vi "hysteresis_fxp_16_5.vi"(8 "N_hyst":u8=3, 11 "uk_in":fxp<+/-,16,5>) -> (3 "Hinv(uk)":fxp<+/-,32,10>)   [LabVIEW 2017]
uses:
  <vilib>/Platform/TimedLoop/XDataNode/timing_clust.ctl
  <vilib>/Platform/TimedLoop/XDataNode/nitl_modes.ctl
  <vilib>/Platform/TimedLoop/XDataNode/wakeup.ctl
  <vilib>/rvi/Emulation/niFpgaSctlEmulationGetInTimedLoop.vi
  <vilib>/rvi/Emulation/niFpgaEmulationReportErrorSimple.vi
  <vilib>/rvi/Emulation/niFpgaGetClockAttributes.vi
  <vilib>/rvi/Emulation/niFpgaCriticalErrorInLSC.vi
  <vilib>/rvi/Memory/Memory_Emulation/nirvimemoryFastEmulation.vi
  <vilib>/rvi/Memory/Memory_Emulation/nirvimemoryEmulation.vi
  <vilib>/rvi/Emulation/niFpgaEmulationIsFPGAContextNoSignature.vi
  <vilib>/rvi/DataTransferAndStorage/Container/Common/niFpgaContainerGetUniqueNameForEmu.vi
  <vilib>/rvi/Emulation/niFpgaProcessEmulError.vi
  <vilib>/rvi/errors/nirviReportUnexpectedCaseInternalError (U32).vi
  <vilib>/Platform/TimedLoop/XDataNode/XDataNode.xnode
  <vilib>/rvi/DataTransferAndStorage/Container/XNode/niFpgaContainer.xnode
  <vilib>/rvi/FXPMathLib/FxpSub/XNode/nifxpmath_Sub.xnode
  <vilib>/rvi/FXPMathLib/FxpAdd/XNode/nifxpmath_Add.xnode
  <vilib>/Platform/TimedLoop/XDataNode/XDNodeRunTimeDep.lvlib
  <vilib>/rvi/FXPMathLib/sim/FxpSim.dll
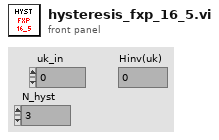
[diagram p1: front panel]
types:
  T1 = typedef "XDNodeRunTimeDep.lvlib/timing_clust.ctl" = cluster{"Expected End [f-1]":u64, "Actual End [f-1]":u64, "Finished Late? [f-1]":bool, "Expected End [i-1]":u64, "Actual End [i-1]":u64, "Finished Late? [i-1]":bool, "Expected Start [i]":u64, "Actual Start [i]":u64, "Expected Start [f]":u64, "Actual Start [f]":u64, "Source Name":string, "Structure Name":string, "Period":i64, "Deadline":i64, "Offset":i64, "Start":i64, "Priority":i32, "Timeout":i32, "Mode":T2, "Wakeup Reason":T3, "Error":errorcluster, "Source Type":string, "Secondary Source Type":string, "Global End Time":u64, "Global Start Time":u64, "Frame Duration":u64, "Iteration Duration":u64, "Assigned CPU":i32, "I/O Scan Engine Mode":u32}
  T2 = typedef "XDNodeRunTimeDep.lvlib/nitl_modes.ctl" = enum32{"No Change", "Process missed periods, maintain original phase", "Discard missed periods, maintain original phase", "Process missed periods, ignore original phase", "Discard missed periods, ignore original phase"}
  T3 = typedef "XDNodeRunTimeDep.lvlib/wakeup.ctl" = enum32{"Normal", "Aborted", "Asynchronous wakeup", "Timing source error", "Timed loop error", "Timeout"}
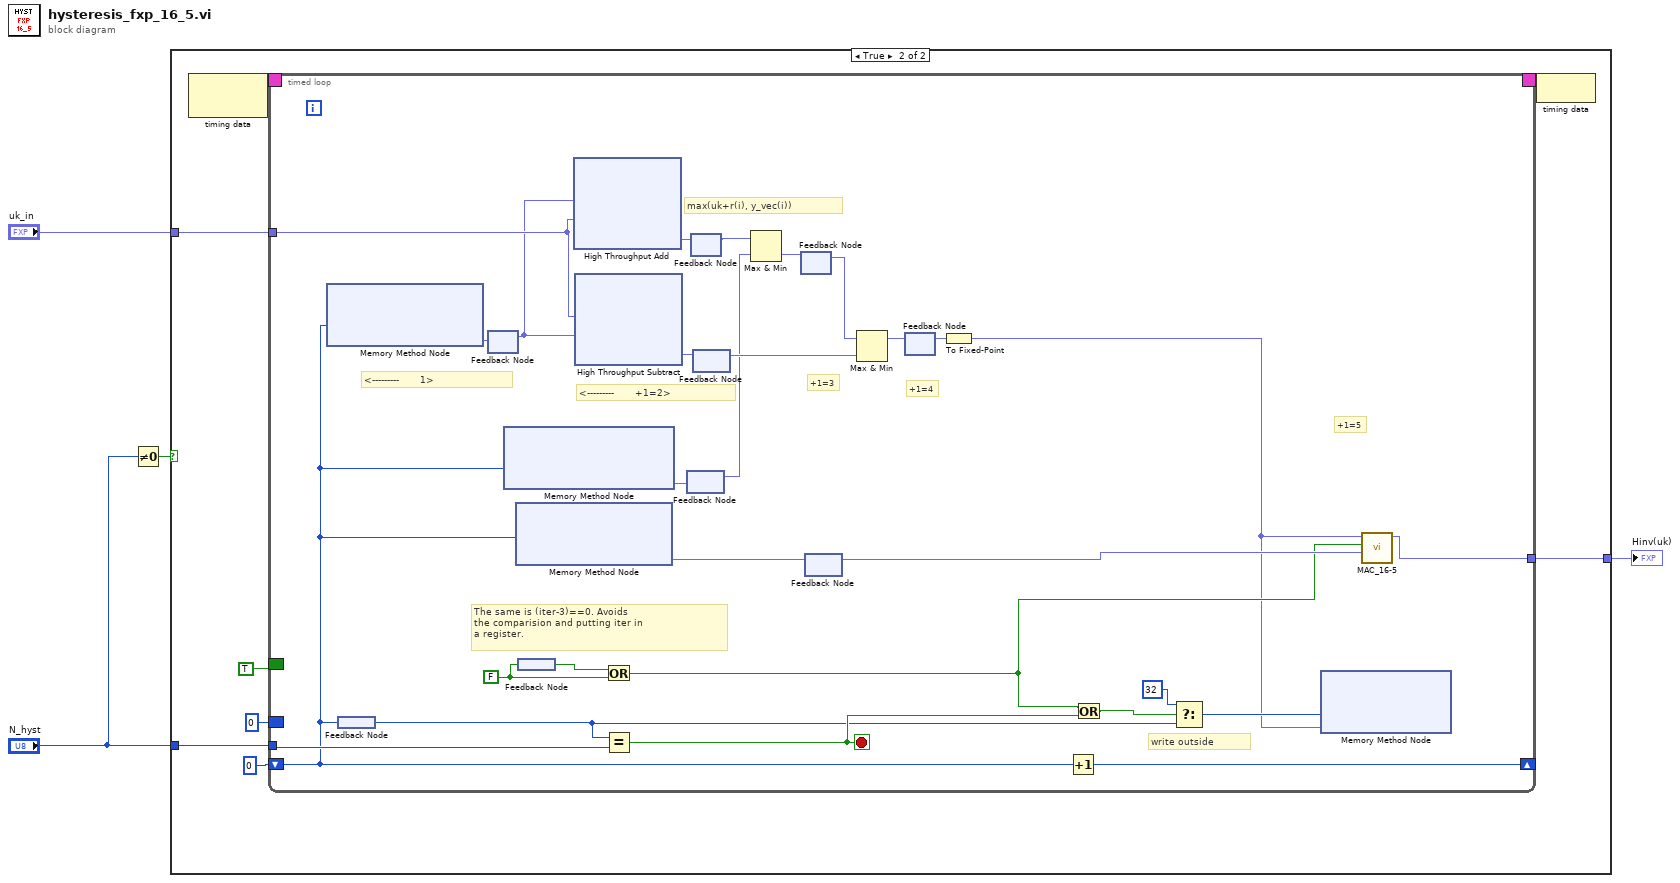
[diagram p0: block diagram]
diagram:
  n1 = Not Equal To 0?(x="N_hyst") -> (x != 0?=w2:bool)
  n2 = case shown="True" w2 {
    tunnel: "N_hyst" -> [_ w9]
    tunnel: "uk_in" -> [w5 w7]
    tunnel: [w5 w6] -> w3
    frame False {
    }
    frame True {
      n3 = node-c288() -> (w13:T1)  [unwired: 1 in]
      n4 = timed-loop {
        timing: w13 -> [_]
        timing-out: [_] -> w12
        tunnel: w7 -> [w41]
        border: u8 0 -> [_]
        tunnel: w9 -> [w36]
        shift-right: [w22] -> _
        shift-left: u8 0 -> [w21]
        border: TRUE -> [_]
        tunnel: [w15] -> w6
        stop <- w26 stop-if-true
        w18 = FALSE
        # "The same is (iter-3)==0. Avoids \nthe comparision and putting iter in \na register."
        # "write outside"
        # "+1=5"
        # "<---------       +1=2>"
        # "+1=4"
        # "+1=3"
        # "<---------       1>"
        # "max(uk+r(i), y_vec(i))"
        n5 = xnode ("Memory Method Node")("Address"=w21) -> ("Data"=w25:fxp<+/-,16,5>)  [unwired: 1 in, 1 out]
        n6 = feedback #1() -> (w20:u8)
        n7 = feedback-in #1(w21) -> ()
        n8 = feedback #2() -> (w24:fxp<+/-,16,5>)  [unwired: 1 in]
        n9 = feedback-in #2(w25) -> ()
        n10 = xnode ("Memory Method Node")("Address"=w21) -> ("Data"=w31:fxp<+/-,16,5>)  [unwired: 1 in, 1 out]
        n11 = xnode ("Memory Method Node")("Address"=w21) -> ("Data"=w23:fxp<+/-,16,5>)  [unwired: 1 in, 1 out]
        n12 = feedback #3() -> (w19:bool)
        n13 = feedback-in #3(w18) -> ()
        n14 = xnode ("High Throughput Add")("x"=w24, "y"=w41) -> ("x+y"=w39:fxp<+/-,17,6>)
        n15 = xnode "High Throughput Subtract"("x"=w41, "y"=w24) -> ("x-y"=w38:fxp<+/-,17,6>)
        n16 = Or(x=w19, y=w18) -> (x .or. y?=w16:bool)
        n17 = Equal?(x=w20, y=w36) -> (x = y?=w26:bool)
        n18 = feedback #4() -> (w30:fxp<+/-,16,5>)  [unwired: 1 in]
        n19 = feedback-in #4(w31) -> ()
        n20 = feedback-in #5(w39) -> ()
        n21 = feedback #5() -> (w40:fxp<+/-,17,6>)  [unwired: 1 in]
        n22 = feedback #6() -> (w32:fxp<+/-,17,6>)  [unwired: 1 in]
        n23 = feedback-in #6(w38) -> ()
        n24 = Max & Min(x=w40, y=w30) -> (min(x,y)=w37:fxp<+/-,17,6>)  [unwired: 1 out]
        n25 = feedback #7() -> (w34:fxp<+/-,17,6>)  [unwired: 1 in]
        n26 = feedback-in #7(w37) -> ()
        n27 = feedback #8() -> (w17:fxp<+/-,16,5>)  [unwired: 1 in]
        n28 = feedback-in #8(w23) -> ()
        n29 = Max & Min(x=w34, y=w32) -> (max(x,y)=w35:fxp<+/-,17,6>)  [unwired: 1 out]
        n30 = feedback #9() -> (w33:fxp<+/-,17,6>)  [unwired: 1 in]
        n31 = feedback-in #9(w35) -> ()
        n32 = To Fixed-Point(number=w33) -> (fixed-point=w14:fxp<+/-,16,5>)  [unwired: 1 in]
        n33 = Increment(x=w21) -> (x+1=w22:u8)
        n34 = Or(x=w16, y=w26) -> (x .or. y?=w27:bool)
        n35 = Select(t=u8 32, s=w27, f=w20) -> (s? t:f=w29:u8)
        n36 = xnode ("Memory Method Node")("Address"=w29, "Data"=w14) -> ()  [unwired: 1 in, 1 out]
        n37 = call "MAC_16-5.vi"("b"=w17, "sclr"=w16, "a"=w14) -> ("s"=w15:fxp<+/-,32,10>)  [unwired: 8 in]
      }
      n38 = node-c288(w12) -> ()
    }
  }
  "Hinv(uk)" <- w3
